vi "generate_footer.vi"() -> (0 "footer":string)   [LabVIEW 2024]
uses:
  <userlib>/_OpenG.lib/md5/md5.llb/MD5 Message Digest (Hexadecimal String)__ogtk.vi
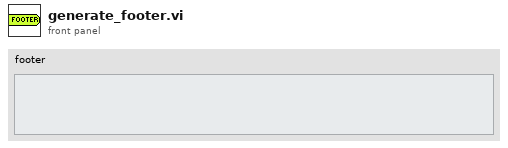
[diagram p1: front panel]
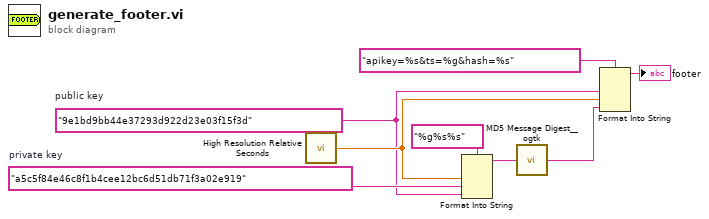
[diagram p0: block diagram]
diagram:
  w1 = "9e1bd9bb44e37293d922d23e03f15f3d"  # public key
  w2 = "a5c5f84e46c8f1b4cee12bc6d51db71f3a02e919"  # private key
  n1 = call <vilib>:"High Resolution Relative Seconds.vi"() -> ("relative seconds"=w3:dbl)
  n2 = Format Into String(format string="%g%s%s", w3, w2, w1) -> (resulting string=w6:string)  [unwired: 2 in, 1 out]
  n3 = call-poly <userlib>:"MD5 Message Digest__ogtk.vi"("Message"=w6) -> ("MD5 Message Digest"=w5:string)
  n4 = Format Into String(format string="apikey=%s&ts=%g&hash=%s" ("public key"), w1, w3, w5) -> (resulting string=→"footer":string)  [unwired: 2 in, 1 out]
